vi "time.vi"() -> ()   [LabVIEW 2021]
panel:
  out "output 1":timestamp format="%<%H:%M:%S\n%d/%m/%Y>T"
  out "date/time string":string
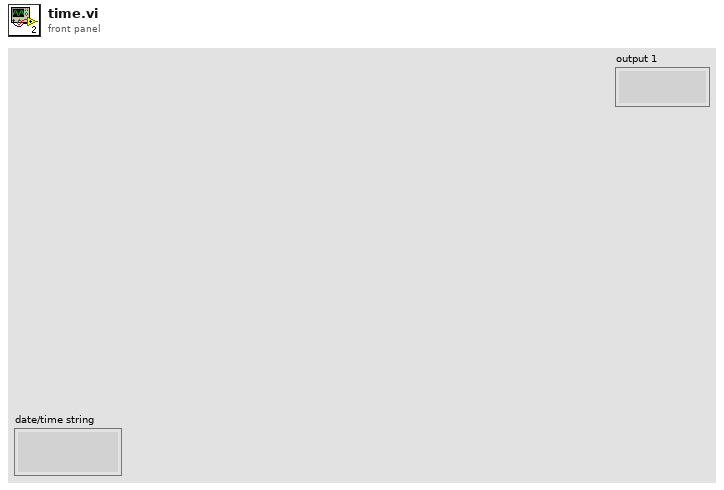
[diagram p1: front panel]
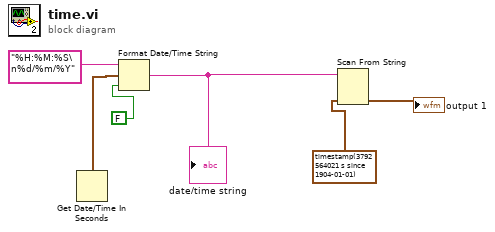
[diagram p0: block diagram]
diagram:
  n1 = Get Date/Time In Seconds() -> (seconds since 1Jan1904=w6:timestamp)
  n2 = Format Date/Time String(time format string (%c)="%H:%M:%S\n%d/%m/%Y", seconds (now)=w6, UTC format=FALSE) -> (date/time string=w5:string)
  "date/time string" <- w5
  n3 = Scan From String "Scan From String"(input string=w5, default 1=timestamp(3792564021.548434 s since 1904-01-01)) -> (output 1=→"output 1":timestamp)  [unwired: 3 in, 3 out]
